vi "Constructor.vi"(8 "error in (no error)":errorcluster, 10 "Fit Controls":T1={"Pre-peak-ms"=30.0, "Onset threshold (%)"=4.0, "Window size (+- ms)"=5.0, "Window Centres\n(ms after onset)"=[20.0, 40.0, 60.0]}, 11 "Sample Rate":i32) -> (0 "error out":errorcluster, 3 "Head Impulse Fit out":refnum<class "Head Impulse Fit.lvclass">)   [LabVIEW 2014, in "Head Impulse Fit.lvclass"]
uses:
  Head Impulse Fit.lvclass
  Fit Controls.ctl
  Head Impulse Fit.lvclass/Head Impulse Fit.ctl
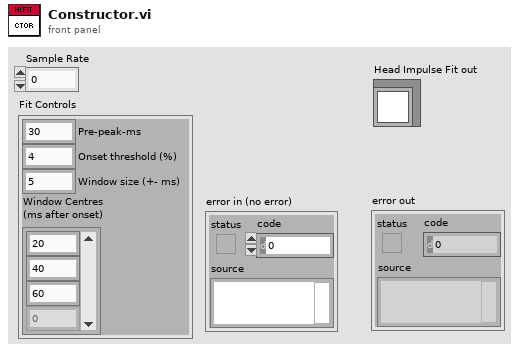
[diagram p1: front panel]
types:
  T1 = typedef "Head Impulse Fit.lvclass/Fit Controls.ctl" = cluster{"Pre-peak-ms":dbl, "Onset threshold (%)":dbl, "Window size (+- ms)":dbl, "Window Centres\n(ms after onset)":dbl[]}
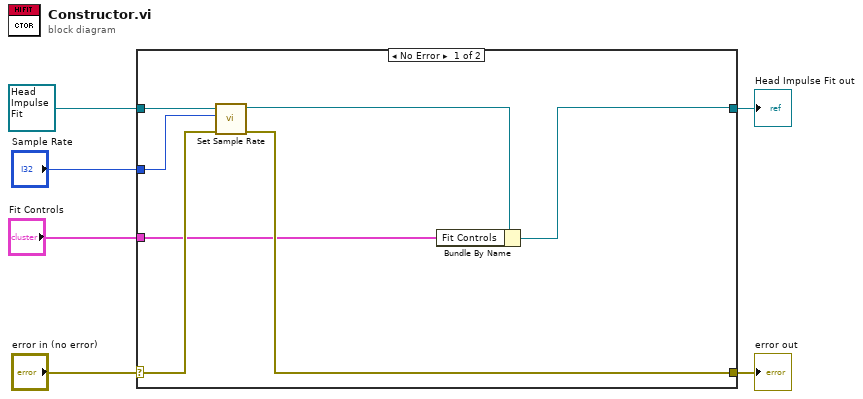
[diagram p0: block diagram]
diagram:
  n1 = case shown="No Error" "error in (no error)" {
    selector: "error in (no error)" -> [w11 w15]
    tunnel: [w10 w15] -> w5
    tunnel: [w8 w14] -> w4
    tunnel: refnum<class "Head Impulse Fit.lvclass"> refnum ("Head Impulse Fit.lvclass") -> [w13 w14]
    tunnel: "Sample Rate" -> [w12 _]
    tunnel: "Fit Controls" -> [w7 _]
    frame No Error {
      n2 = call-dynamic "Set Sample Rate.vi"("error in (no error)"=w11, "Sample Rate"=w12, "Abstract Fit in"=w13) -> ("error out"=w10:errorcluster, "Abstract Fit out"=w9:refnum<class "Head Impulse Fit.lvclass">)  [unwired: 7 in]
      n3 = Bundle By Name(cluster=w9, "Fit Controls"=w7) -> (w8:refnum<class "Head Impulse Fit.lvclass">)
    }
    frame Error {
    }
  }
  "error out" <- w5
  "Head Impulse Fit out" <- w4
